vi "CalcTime.vi"(0 "TickRef":refnum<k21>, 5 "TockRef":refnum<k21>, 11 "resetMaxTime":bool) -> (4 "Time":u32, 6 "MaxTime":u32)   [LabVIEW 2015, in "Timers.lvlib"]
uses:
  Timers.lvlib
  <vilib>/rvi/DataTransferAndStorage/Container/Common/niFpgaContainerExecOnDevCompGetState.vi
  <vilib>/rvi/Emulation/niFpgaEmulationIsFPGAContextNoSignature.vi
  <vilib>/rvi/DataTransferAndStorage/Container/Common/niFpgaContainerGetUniqueNameForEmu.vi
  <vilib>/rvi/Memory/Memory_Emulation/niFpgaMemoryEmulationCacheClearOnFirstRun.vi
  <vilib>/rvi/Memory/Memory_Emulation/nirvimemoryEmulationManagerCache_MakeExclusive.vi
  <vilib>/rvi/Memory/Memory_Emulation/niFpgaMemoryEmulationValidateCache.vi
  <vilib>/rvi/Memory/Memory_Emulation/nirvimemoryEmulationManagerCache_InsertValue.vi
  <vilib>/Utility/error.llb/Clear Errors.vi
  <vilib>/rvi/Memory/Memory_Emulation/nirvimemoryEmulationManagerCache_ReleaseExclusive.vi
  <vilib>/rvi/Memory/Memory_Emulation/nirvimemoryEmulationManagerCache_GetValue.vi
  <vilib>/rvi/Memory/Memory_Emulation/nirvimemoryEmulationManagerCache_SetValue.vi
  <vilib>/rvi/Emulation/niFpgaProcessEmulError.vi
  <vilib>/rvi/Emulation/niFpgaSctlEmulationGetInTimedLoop.vi
  <vilib>/rvi/DataTransferAndStorage/Container/XNode/niFpgaContainer.xnode
  <vilib>/rvi/DataTransferAndStorage/Register/Emulation/niFpgaRegisterEmulationRefIn.vi
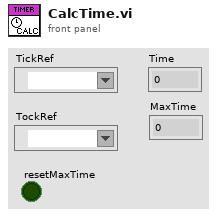
[diagram p1: front panel]
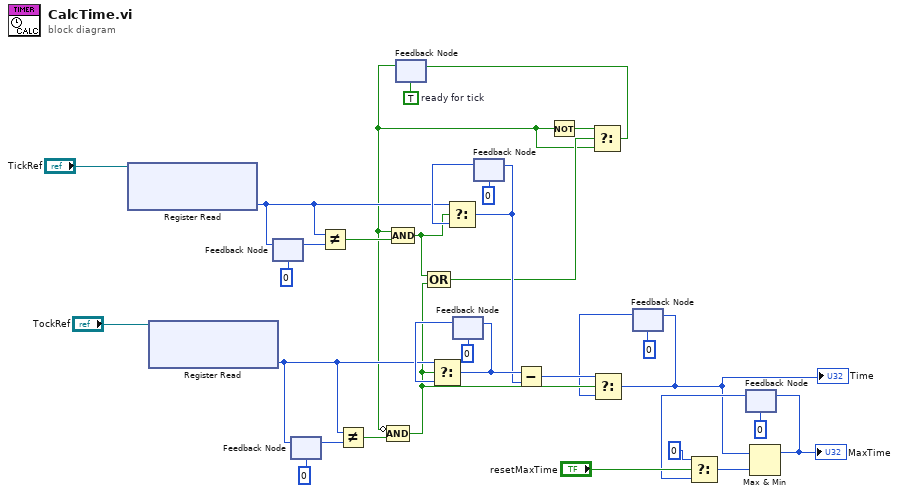
[diagram p0: block diagram]
diagram:
  w19 = TRUE  # ready for tick
  n1 = xnode ("Register Read")("Register In"="TickRef") -> ("Data"=w18:u32)  [unwired: 1 out]
  n2 = xnode ("Register Read")("Register In"="TockRef") -> ("Data"=w12:u32)  [unwired: 1 out]
  n3 = feedback-in #1(w18) -> ()
  n4 = feedback #1(u32 0 ("Data")) -> (w16:u32)
  n5 = feedback #2(u32 0 ("Data")) -> (w14:u32)
  n6 = feedback-in #2(w12) -> ()
  n7 = Not Equal?(x=w18, y=w16) -> (x != y?=w15:bool)
  n8 = Not Equal?(x=w12, y=w14) -> (x != y?=w11:bool)
  n9 = feedback #3(w19) -> (w7:bool)
  n10 = Compound Arithmetic op=AND(invert w7, w11) -> (w4:bool)
  n11 = Compound Arithmetic op=AND(w7, w15) -> (w10:bool)
  n12 = Compound Arithmetic op=OR(w10, w4) -> (w9:bool)
  n13 = feedback #4(u32 0 ("Data")) -> (w29:u32)
  n14 = Select(t=w12, s=w4, f=w29) -> (s? t:f=w27:u32)
  n15 = feedback-in #4(w27) -> ()
  n16 = feedback #5(u32 0 ("Data")) -> (w30:u32)
  n17 = Select(t=w18, s=w10, f=w30) -> (s? t:f=w26:u32)
  n18 = feedback-in #5(w26) -> ()
  n19 = Subtract(x=w27, y=w26) -> (x-y=w3:u32)
  n20 = Not(x=w7) -> (.not. x?=w8:bool)
  n21 = Select(t=w8, s=w9, f=w7) -> (s? t:f=w6:bool)
  n22 = feedback-in #3(w6) -> ()
  n23 = feedback #6(u32 0 ("Data")) -> (w2:u32)
  n24 = Select(t=w3, s=w4, f=w2) -> (s? t:f=w1:u32)
  "Time" <- w1
  n25 = feedback-in #6(w1) -> ()
  n26 = feedback #7(u32 0 ("MaxTime")) -> (w23:u32)
  n27 = Select(t=u32 0, s="resetMaxTime", f=w23) -> (s? t:f=w22:u32)
  n28 = Max & Min(x=w1, y=w22) -> (max(x,y)=w21:u32)  [unwired: 1 out]
  "MaxTime" <- w21
  n29 = feedback-in #7(w21) -> ()
